vi "serial_a0.vi"(0 "VISA resource name":refnum<visa-resource-name>="COM1", 1 "baud rate":u32=9600, 2 "data bits":u16=8 min=5 max=8 step=1, 3 "parity":u16(ring) items=["None", "Odd", "Even", "Mark", "Space"], 4 "stop bits":u16(ring)=10 items=["1.0"=10, "1.5"=15, "2.0"=20], 5 "write":bool=TRUE, 6 "read":bool=TRUE, 7 "flow control":u16(ring) items=["None"=0, "XON/XOFF"=1, "RTS/CTS"=2, "DTR/DSR"=4], 8 "string to write":string="A0") -> (9 "read string":string, 10 "bytes read":u32)   [LabVIEW 2009]
doc: "The Basic Serial Read and Write example performs a Serial Port Read, a Serial Port Write, or a combination of these actions. The user selects the actions (read or write) on the front panel. If both are selected, the VI will write the data first, read data, and then close the VISA session that is opened to the port. This VI will wait until the specified number of bytes is received at the port. Only the number of bytes specified will be read.\n\nINSTRUCTIONS:\n1) Select the serial resource and configuration parameters (baud rate, data bits, parity, stop bits, flow control).\n2) Select the operations to be performed. \n3) Connect the serial port to your device. If no device is available, perform a loopback test by doing one of the following. Short pins 2 and 3 on a RS-232 cable or short pin 4 to pin 8 and pin 5 to pin 9 on a RS-485/422 cable. \n4) Run the VI to see the data read. (The \"read string\" will match the \"string to write\" if a loopback test was performed.)\n\nNote: The parameters set for the serial port must match the parameters of the connected instrument or device. In this example, the bytes to read parameter specifies the number of bytes that the serial port reads. If there were more bytes at the port than the number specified in bytes to read, those bytes would not be read. Also, if you specify to read more bytes than the number of bytes actually read, you might receive a timeout error message.\n\nOn the block diagram, the Configure Serial Port VI sets the configuration parameters. The front panel displays the controls used to configure the basic parameters, such as baud rate, data bits, and parity. Constants configure the other parameters the user probably does not need set. After the VISA Configure Serial Port VI opens the VISA session and configures the port, the VI passes the VISA resource name to other VIs that perform operations on that VISA resource. The VISA Write function sends a command to the serial device and the VISA Read function returns data based on the command. The VISA Close function then closes the reference to the serial device. It is important to close the reference; otherwise communication through with that port through protocols other than VISA might not be possible."
uses:
  <vilib>/Instr/_visa.llb/VISA Configure Serial Port (Instr).vi
panel:
  out "Meter":dbl(knob) scale=0.0..1024.0
  out "Grafic":i32(graph)
  out "Numeric":i32
  in  "delay before read (ms)":u32=5
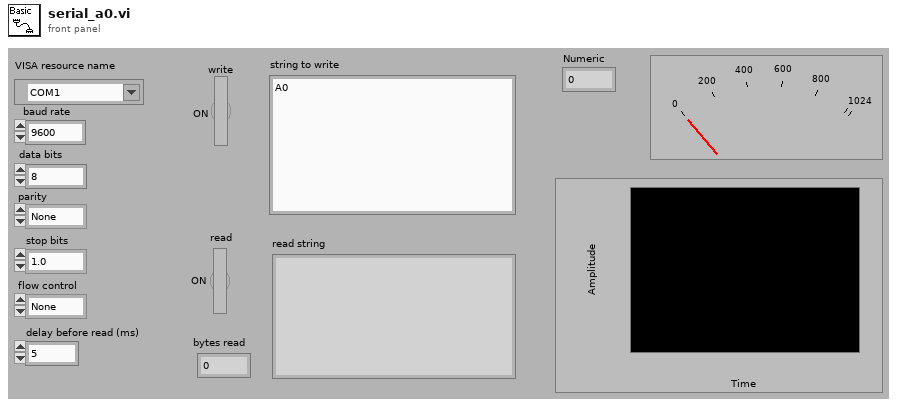
[diagram p1: front panel]
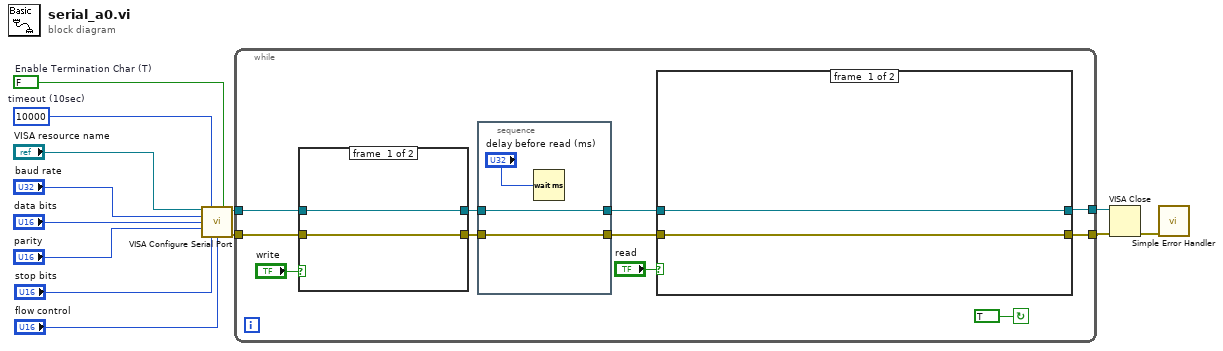
[diagram p0: block diagram]
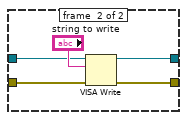
[diagram p2: hidden frame]
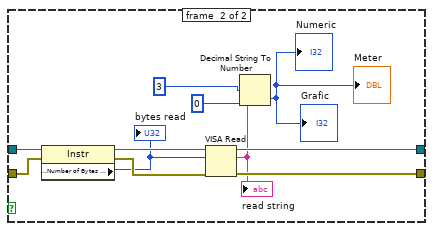
[diagram p3: hidden frame]
diagram:
  w4 = FALSE  # Enable Termination Char (T)
  w5 = u32 10000  # timeout (10sec)
  n1 = call-poly "VISA Configure Serial Port"("VISA resource name"="VISA resource name", "timeout (10sec)"=w5, "Enable Termination\nChar (T)"=w4, "baud rate (9600)"="baud rate", "data bits (8)"="data bits", "parity (0:none)"="parity", "stop bits (10: 1 bit)"="stop bits", "flow control (0:none)"="flow control") -> ("VISA resource name out"=w10:refnum<visa-resource-name>, "error out"=w11:errorcluster)  [unwired: 1 in, 5 out]
  n2 = while {
    tunnel: w11 -> [w23]
    tunnel: w10 -> [w22]
    tunnel: [w21] -> w9
    tunnel: [w20] -> w8
    stop <- TRUE continue-if-true
    n3 = case shown="True" "write" {
      tunnel: [w29 w34] -> w18
      tunnel: w22 -> [w28 w32]
      tunnel: w23 -> [w29 w31]
      tunnel: [w28 w30] -> w16
      frame #0 {
      }
      frame #1 {
        n4 = VISA Write(VISA resource name=w32, write buffer="string to write", error in (no error)=w31) -> (VISA resource name out=w30:refnum<visa-resource-name>, error out=w34:errorcluster)  [unwired: 1 out]
      }
    }
    n5 = stacked-sequence {
      tunnel: w18 -> [w27]
      tunnel: [w27] -> w17
      tunnel: w16 -> [w26]
      tunnel: [w26] -> w15
      frame #0 {
        n6 = Wait (ms)(milliseconds to wait="delay before read (ms)") -> ()  [unwired: 1 out]
      }
    }
    n7 = case shown="True" "read" {
      tunnel: w17 -> [w36 w43]
      tunnel: [w36 w47] -> w21
      tunnel: [w35 w46] -> w20
      tunnel: w15 -> [w35 w45]
      frame #0 {
      }
      frame #1 {
        n8 = property class="Instr"(reference=w45, error in=w43) -> (reference out=w44:refnum<visa-resource-name>, error out=w42:errorcluster, "Serial Settings:Number of Bytes at Serial Port"=w41:u32)
        "bytes read" <- w41
        n9 = VISA Read(VISA resource name=w44, byte count=w41, error in (no error)=w42) -> (VISA resource name out=w46:refnum<visa-resource-name>, read buffer=w40:string, error out=w47:errorcluster)  [unwired: 1 out]
        "read string" <- w40
        n10 = Decimal String To Number(string=w40, offset=3, default (0L)=0) -> (number=→"Numeric" →"Grafic" →"Meter":i32)  [unwired: 1 out]
      }
    }
  }
  n11 = VISA Close(VISA resource name=w8, error in (no error)=w9) -> (error out=w7:errorcluster)
  n12 = call <vilib>:"Simple Error Handler.vi"("error in (no error)"=w7) -> ()  [unwired: 1 in, 8 out]
